vi "SetAttn.vi"(11 "Attenuation":u8(slide) scale=0.0..63.0) -> (0 "error out":errorcluster)   [LabVIEW 2022 SP3]
uses:
  <vilib>/DAQmx/write.llb/DAQmx Write (Digital 1D U8 NChan 1Samp).vi
  <vilib>/DAQmx/miscellaneous.llb/DAQmx Fill In Error Info.vi
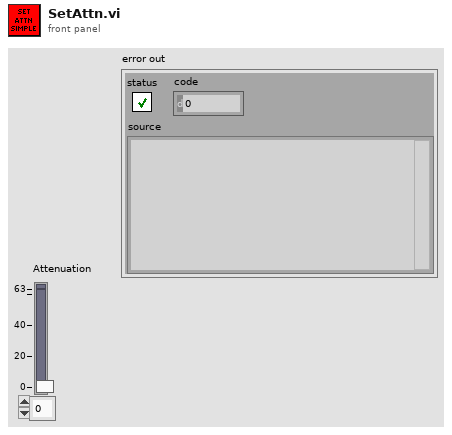
[diagram p1: front panel]
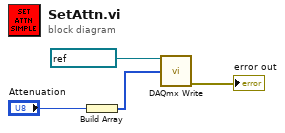
[diagram p0: block diagram]
diagram:
  n1 = Build Array("Attenuation") -> (w2:u8[])
  n2 = call-poly <vilib>:"DAQmx Write.vi"("task/channels in"=refnum<k21> "Hitachi", "data"=w2) -> ("error out"=→"error out":errorcluster)  [unwired: 11 in, 2 out]
